vi "FTW-JSON-Format-Path.vi"(1 "LabVIEW Path":path) -> (0 "JSON String":string)   [LabVIEW 2013]
panel:
  # "Inputs"
  # "Outputs"
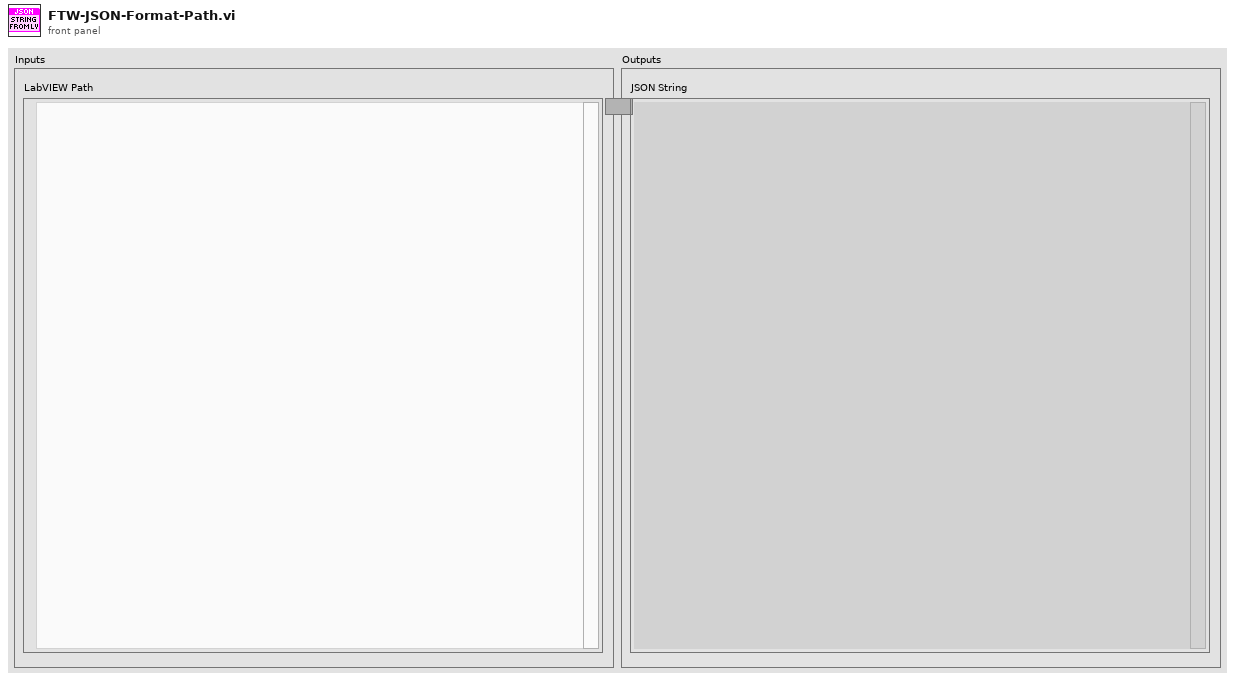
[diagram p1: front panel]
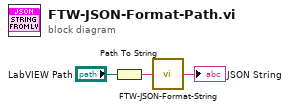
[diagram p0: block diagram]
diagram:
  n1 = Path To String(path="LabVIEW Path") -> (string=w1:string)
  n2 = call "FTW-JSON-Format-String.vi"("LabVIEW String"=w1) -> ("JSON String"=→"JSON String":string)
